vi "DELETE In-Place Debug.vi"   [LabVIEW 2013]
uses:
  Action.ctl
types:
  T1 = typedef "Action.ctl" = enum16{"GET", "PUT", "DELETE"}
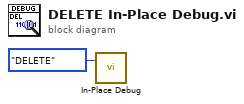
[diagram p0: block diagram]
diagram:
  n1 = call "In-Place Debug.vi"("Action"=Action."DELETE") -> ()  [unwired: 2 in, 1 out]
